vi "Robot_info_to-from_dash.vi"() -> ()   [LabVIEW 2015]
uses:
  Robot Global Data.vi
panel:
  out "error":errorcluster
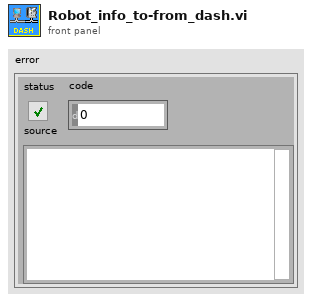
[diagram p1: front panel]
types:
  T1 = cluster{"Record?":bool, "Current File":string, "Run script?":bool, "Stop recording?":bool, "Stop script?":bool}
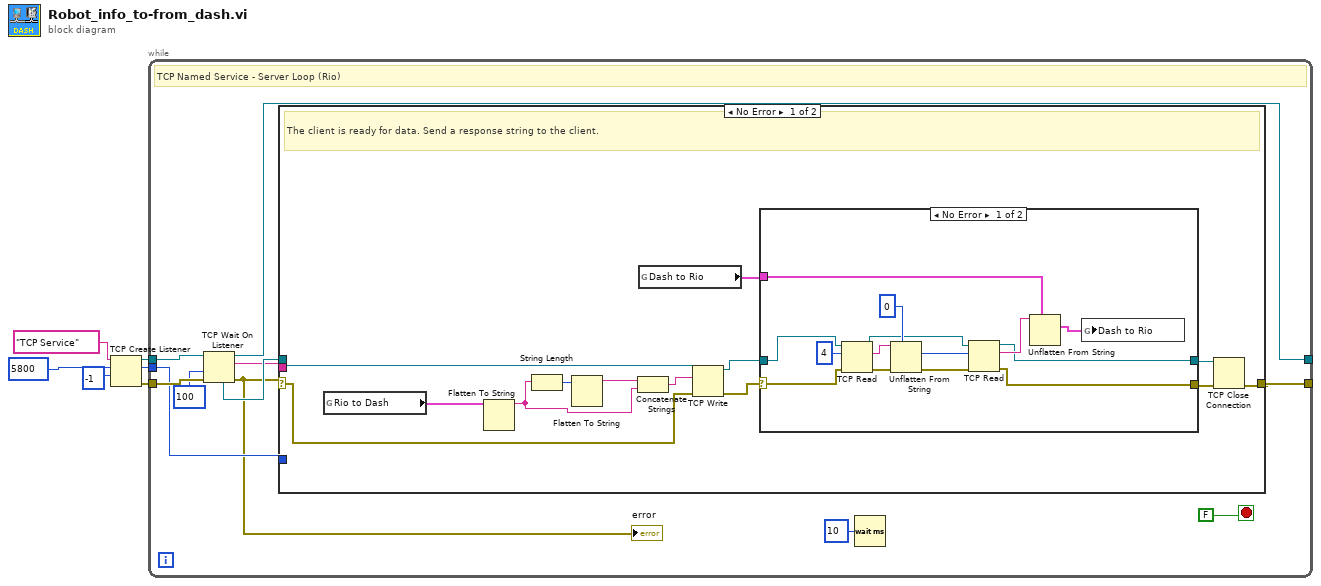
[diagram p0: block diagram]
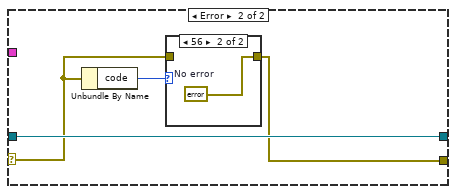
[diagram p2: hidden frame]
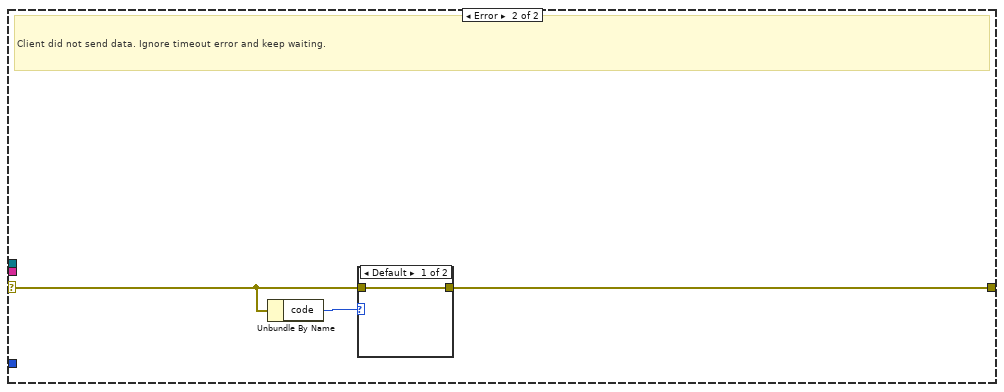
[diagram p4: hidden frame]
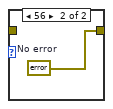
[diagram p5: hidden frame]
diagram:
  n1 = TCP Create Listener(9:-1 ("timeout ms (25000)"), 10:u16 5800 ("port"), 11:"TCP Service" ("service name")) -> (0:w4:errorcluster, 2:w5:u16, 3:w6:refnum<k5>)  [unwired: 2 in]
  n2 = while {
    tunnel: [w13] -> _
    tunnel: w6 -> [w17]
    tunnel: w4 -> [w16]
    tunnel: [w10] -> _
    tunnel: w5 -> [w14]
    stop <- FALSE ("Stop") stop-if-true
    # "TCP Named Service - Server Loop (Rio)"
    n3 = TCP Wait On Listener(8:w16, 9:100 ("timeout ms (25000)"), 11:w17) -> (0:w8:errorcluster, 2:w11:string, 3:w10:refnum<k5>, 4:w15:refnum<k5>)  [unwired: 1 in, 1 out]
    "error" <- w8
    n4 = case shown="No Error" w8 {
      selector: w8 -> [w21 w53]
      tunnel: [w30 w51] -> w13
      tunnel: w15 -> [w25 _]
      tunnel: w14 -> [_ _]
      tunnel: w11 -> [_ _]
      frame No Error {
        # "The client is ready for data. Send a response string to the client."
        n5 = global read "Robot Global Data.vi" "Rio to Dash"() -> (w18:cluster{"Recording?":bool, "Running?":bool})
        n6 = Flatten To String(anything=w18) -> (data string=w29:string)  [unwired: 3 in, 2 out]
        n7 = String Length(string=w29) -> (length=w27:i32)
        n8 = Flatten To String(anything=w27) -> (data string=w28:string)  [unwired: 3 in, 2 out]
        n9 = Concatenate Strings(w28, w29) -> (w24:string)
        n10 = global read "Robot Global Data.vi" "Dash to Rio"() -> (w26:T1)
        n11 = TCP Write(connection ID=w25, data in=w24, error in (no error)=w21) -> (connection ID out=w19:refnum<k5>, error out=w20:errorcluster)  [unwired: 1 in, 1 out]
        n12 = case shown="No Error" w20 {
          selector: w20 -> [w33 w46]
          tunnel: w26 -> [w44 _]
          tunnel: [w35 w45] -> w23
          tunnel: [w34 w48] -> w22
          tunnel: w19 -> [w32 w48]
          frame No Error {
            n13 = TCP Read(connection ID=w32, bytes to read=4, error in (no error)=w33) -> (connection ID out=w37:refnum<k5>, data out=w41:string, error out=w42:errorcluster)  [unwired: 2 in]
            n14 = Unflatten From String(type=0, binary string=w41, error in (no error)=w42) -> (value=w38:i32, error out=w39:errorcluster)  [unwired: 2 in, 1 out]
            n15 = TCP Read(connection ID=w37, bytes to read=w38, error in (no error)=w39) -> (connection ID out=w34:refnum<k5>, data out=w36:string, error out=w35:errorcluster)  [unwired: 2 in]
            n16 = Unflatten From String(type=w44, binary string=w36) -> (value=w31:T1)  [unwired: 3 in, 2 out]
            n17 = global write "Robot Global Data.vi" "Dash to Rio"(w31) -> ()
          }
          frame Error {
            n18 = Unbundle By Name(w46) -> ("code"=w47:i32)
            n19 = case shown="56" w47 {
              tunnel: w46 -> [w49 _]
              tunnel: [w49 w50] -> w45
              frame Default {
              }
              frame 56 {
                w50 = errorcluster {"status"=FALSE, "code"=0, "source"=""}  # No error
              }
            }
          }
        }
        n20 = TCP Close Connection(connection ID=w22, error in (no error)=w23) -> (error out=w30:errorcluster)  [unwired: 1 in, 1 out]
      }
      frame Error {
        # "Client did not send data. Ignore timeout error and keep waiting."
        n21 = Unbundle By Name(w53) -> ("code"=w52:i32)
        n22 = case shown="Default" w52 {
          tunnel: w53 -> [w54 _]
          tunnel: [w54 w55] -> w51
          frame Default {
          }
          frame 56 {
            w55 = errorcluster {"status"=FALSE, "code"=0, "source"=""}  # No error
          }
        }
      }
    }
    n23 = Wait (ms)(milliseconds to wait=u32 10) -> ()  [unwired: 1 out]
  }
